vi "PhiCorrect_RAW.vi"(1 "PhiCorrect_RAW":i16=773, 2 "RAW cmds 2D in":i16[][](array[numeric])=[[-21913, -13120, -6560, 0, 4372, 4384, -21862, -1, -21913, -13120, -6560, 0, 4328, 4340, -21862, -1, -21913, -13120, -6560, 0, 4284, 4296, -21862, -1, -21913, -13120, -6560, 0, 4240, 4251, -21862, -1, -21913, -13120, -6560, 0, 4195, 4207, -21862, -1, -21913, -13120, -6560, 0, 4151, 4163, -21862, -1, -21913, -13120, -6560, 0, 4107, 4118, -21862, -1, -21913, -13120, -6560, 0, 4063, 4074, -21862, -1, -21913, -13120, -6560, 0, 4019, 4030, -21862, -1, -21913, -13120, -6560, 0, 3975, 3986, -21862, -1, -21913, -13120, -6560, 0, 3930, 3941, -21862, -1, -21913, -13120, -6560, 0, 3886, 3897, -21862, -1, -21913, -13120, -6560, 0, 3842, 3853, -21862, -1, -21913, -13120, -6560, 0, 3798, 3808, -21862, -1, -21913, -13120, -6560, 0, 3754, 3764, -21862, -1, -21913, -13120, -6560, 0, 3710, 3720, -21862, -1, -21913, -13120, -6560, 0, 3665, 3675, -21862, -1, -21913, -13120, -6560, 0, 3621, 3631, -21862, -1, -21913, -13120, -6560, 0, 3577, 3587, -21862, -1, -21913, -13120, -6560, 0, 3533, 3543, -21862, -1, -21913, -13120, -6560, 0, 3489, 3498, -21862, -1, -21913, -13120, -6560, 0, 3444, 3454, -21862, -1, -21913, -13120, -6560, 0, 3400, 3410, -21862, -1, -21913, -13120, -6560, 0, 3356, 3365, -21862, -1, -21913, -13120, -6560, 0, 3312, 3321, -21862, -1, -21913, -13120, -6560, 0, 3268, 3277, -21862, -1, -21913, -13120, -6560, 0, 3224, 3233, -21862, -1, -21913, -13120, -6560, 0, 3179, 3188, -21862, -1, -21913, -13120, -6560, 0, 3135, 3144, -21862, -1, -21913, -13120, -6560, 0, 3091, 3100, -21862, -1, -21913, -13120, -6560, 0, 3047, 3055, -21862, -1, -21913, -13120, -6560, 0, 3003, 3011, -21862, -1, -21913, -13120, -6560, 0, 2959, 2967, -21862, -1, -21913, -13120, -6560, 0, 2914, 2922, -21862, -1, -21913, -13120, -6560, 0, 2870, 2878, -21862, -1, -21913, -13120, -6560, 0, 2826, 2834, -21862, -1, -21913, -13120, -6560, 0, 2782, 2790, -21862, -1, -21913, -13120, -6560, 0, 2738, 2745, -21862, -1, -21913, -13120, -6560, 0, 2694, 2701, -21862, -1, -21913, -13120, -6560, 0, 2649, 2657, -21862, -1, -21913, -13120, -6560, 0, 2605, 2612, -21862, -1, -21913, -13120, -6560, 0, 2561, 2568, -21862, -1, -21913, -13120, -6560, 0, 2517, 2524, -21862, -1, -21913, -13120, -6560, 0, 2473, 2479, -21862, -1, -21913, -13120, -6560, 0, 2429, 2435, -21862, -1, -21913, -13120, -6560, 0, 2384, 2391, -21862, -1, -21913, -13120, -6560, 0, 2340, 2347, -21862, -1, -21913, -13120, -6560, 0, 2296, 2302, -21862, -1, -21913, -13120, -6560, 0, 2252, 2258, -21862, -1, -21913, -13120, -6560, 0, 2208, 2214, -21862, -1, -21913, -13120, -6560, 0, 2164, 2169, -21862, -1, -21913, -13120, -6560, 0, 2119, 2125, -21862, -1, -21913, -13120, -6560, 0, 2075, 2081, -21862, -1, -21913, -13120, -6560, 0, 2031, 2037, -21862, -1, -21913, -13120, -6560, 0, 1987, 1992, -21862, -1, -21913, -13120, -6560, 0, 1943, 1948, -21862, -1, -21913, -13120, -6560, 0, 1898, 1904, -21862, -1, -21913, -13120, -6560, 0, 1854, 1859, -21862, -1, -21913, -13120, -6560, 0, 1810, 1815, -21862, -1, -21913, -13120, -6560, 0, 1766, 1771, -21862, -1, -21913, -13120, -6560, 0, 1722, 1726, -21862, -1, -21913, -13120, -6560, 0, 1678, 1682, -21862, -1, -21913, -13120, -6560, 0, 1633, 1638, -21862, -1, -21913, -13120, -6560, 0, 1589, 1594, -21862, -1, -21913, -13120, -6560, 0, 1545, 1549, -21862, -1, -21913, -13120, -6560, 0, 1501, 1505, -21862, -1, -21913, -13120, -6560, 0, 1457, 1461, -21862, -1, -21913, -13120, -6560, 0, 1413, 1416, -21862, -1, -21913, -13120, -6560, 0, 1368, 1372, -21862, -1, -21913, -13120, -6560, 0, 1324, 1328, -21862, -1, -21913, -13120, -6560, 0, 1280, 1284, -21862, -1, -21913, -13120, -6560, 0, 1236, 1239, -21862, -1, -21913, -13120, -6560, 0, 1192, 1195, -21862, -1, -21913, -13120, -6560, 0, 1148, 1151, -21862, -1, -21913, -13120, -6560, 0, 1103, 1106, -21862, -1, -21913, -13120, -6560, 0, 1059, 1062, -21862, -1, -21913, -13120, -6560, 0, 1015, 1018, -21862, -1, -21913, -13120, -6560, 0, 971, 973, -21862, -1, -21913, -13120, -6560, 0, 927, 929, -21862, -1, -21913, -13120, -6560, 0, 883, 885, -21862, -1, -21913, -13120, -6560, 0, 838, 841, -21862, -1, -21913, -13120, -6560, 0, 794, 796, -21862, -1, -21913, -13120, -6560, 0, 750, 752, -21862, -1, -21913, -13120, -6560, 0, 706, 708, -21862, -1, -21913, -13120, -6560, 0, 662, 663, -21862, -1, -21913, -13120, -6560, 0, 618, 619, -21862, -1, -21913, -13120, -6560, 0, 573, 575, -21862, -1, -21913, -13120, -6560, 0, 529, 531, -21862, -1, -21913, -13120, -6560, 0, 485, 486, -21862, -1, -21913, -13120, -6560, 0, 441, 442, -21862, -1, -21913, -13120, -6560, 0, 397, 398, -21862, -1, -21913, -13120, -6560, 0, 352, 353, -21862, -1, -21913, -13120, -6560, 0, 308, 309, -21862, -1, -21913, -13120, -6560, 0, 264, 265, -21862, -1, -21913, -13120, -6560, 0, 220, 220, -21862, -1, -21913, -13120, -6560, 0, 176, 176, -21862, -1, -21913, -13120, -6560, 0, 132, 132, -21862, -1, -21913, -13120, -6560, 0, 87, 88, -21862, -1, -21913, -13120, -6560, 0, 43, 43, -21862, -1, -21913, -13120, -6560, 0, -1, -1, -21862, -1], [-1, -1, -7, -1, 0, 0, 0, 0, -1, -1, -7, -1, 0, 0, 0, 0, -1, -1, -7, -1, 0, 0, 0, 0, -1, -1, -7, -1, 0, 0, 0, 0, -1, -1, -7, -1, 0, 0, 0, 0, -1, -1, -7, -1, 0, 0, 0, 0, -1, -1, -7, -1, 0, 0, 0, 0, -1, -1, -7, -1, 0, 0, 0, 0, -1, -1, -7, -1, 0, 0, 0, 0, -1, -1, -7, -1, 0, 0, 0, 0, -1, -1, -7, -1, 0, 0, 0, 0, -1, -1, -7, -1, 0, 0, 0, 0, -1, -1, -7, -1, 0, 0, 0, 0, -1, -1, -7, -1, 0, 0, 0, 0, -1, -1, -7, -1, 0, 0, 0, 0, -1, -1, -7, -1, 0, 0, 0, 0, -1, -1, -7, -1, 0, 0, 0, 0, -1, -1, -7, -1, 0, 0, 0, 0, -1, -1, -7, -1, 0, 0, 0, 0, -1, -1, -7, -1, 0, 0, 0, 0, -1, -1, -7, -1, 0, 0, 0, 0, -1, -1, -7, -1, 0, 0, 0, 0, -1, -1, -7, -1, 0, 0, 0, 0, -1, -1, -7, -1, 0, 0, 0, 0, -1, -1, -7, -1, 0, 0, 0, 0, -1, -1, -7, -1, 0, 0, 0, 0, -1, -1, -7, -1, 0, 0, 0, 0, -1, -1, -7, -1, 0, 0, 0, 0, -1, -1, -7, -1, 0, 0, 0, 0, -1, -1, -7, -1, 0, 0, 0, 0, -1, -1, -7, -1, 0, 0, 0, 0, -1, -1, -7, -1, 0, 0, 0, 0, -1, -1, -7, -1, 0, 0, 0, 0, -1, -1, -7, -1, 0, 0, 0, 0, -1, -1, -7, -1, 0, 0, 0, 0, -1, -1, -7, -1, 0, 0, 0, 0, -1, -1, -7, -1, 0, 0, 0, 0, -1, -1, -7, -1, 0, 0, 0, 0, -1, -1, -7, -1, 0, 0, 0, 0, -1, -1, -7, -1, 0, 0, 0, 0, -1, -1, -7, -1, 0, 0, 0, 0, -1, -1, -7, -1, 0, 0, 0, 0, -1, -1, -7, -1, 0, 0, 0, 0, -1, -1, -7, -1, 0, 0, 0, 0, -1, -1, -7, -1, 0, 0, 0, 0, -1, -1, -7, -1, 0, 0, 0, 0, -1, -1, -7, -1, 0, 0, 0, 0, -1, -1, -7, -1, 0, 0, 0, 0, -1, -1, -7, -1, 0, 0, 0, 0, -1, -1, -7, -1, 0, 0, 0, 0, -1, -1, -7, -1, 0, 0, 0, 0, -1, -1, -7, -1, 0, 0, 0, 0, -1, -1, -7, -1, 0, 0, 0, 0, -1, -1, -7, -1, 0, 0, 0, 0, -1, -1, -7, -1, 0, 0, 0, 0, -1, -1, -7, -1, 0, 0, 0, 0, -1, -1, -7, -1, 0, 0, 0, 0, -1, -1, -7, -1, 0, 0, 0, 0, -1, -1, -7, -1, 0, 0, 0, 0, -1, -1, -7, -1, 0, 0, 0, 0, -1, -1, -7, -1, 0, 0, 0, 0, -1, -1, -7, -1, 0, 0, 0, 0, -1, -1, -7, -1, 0, 0, 0, 0, -1, -1, -7, -1, 0, 0, 0, 0, -1, -1, -7, -1, 0, 0, 0, 0, -1, -1, -7, -1, 0, 0, 0, 0, -1, -1, -7, -1, 0, 0, 0, 0, -1, -1, -7, -1, 0, 0, 0, 0, -1, -1, -7, -1, 0, 0, 0, 0, -1, -1, -7, -1, 0, 0, 0, 0, -1, -1, -7, -1, 0, 0, 0, 0, -1, -1, -7, -1, 0, 0, 0, 0, -1, -1, -7, -1, 0, 0, 0, 0, -1, -1, -7, -1, 0, 0, 0, 0, -1, -1, -7, -1, 0, 0, 0, 0, -1, -1, -7, -1, 0, 0, 0, 0, -1, -1, -7, -1, 0, 0, 0, 0, -1, -1, -7, -1, 0, 0, 0, 0, -1, -1, -7, -1, 0, 0, 0, 0, -1, -1, -7, -1, 0, 0, 0, 0, -1, -1, -7, -1, 0, 0, 0, 0, -1, -1, -7, -1, 0, 0, 0, 0, -1, -1, -7, -1, 0, 0, 0, 0, -1, -1, -7, -1, 0, 0, 0, 0, -1, -1, -7, -1, 0, 0, 0, 0, -1, -1, -7, -1, 0, 0, 0, 0, -1, -1, -7, -1, 0, 0, 0, 0, -1, -1, -7, -1, 0, 0, 0, 0, -1, -1, -7, -1, 0, 0, 0, 0, -1, -1, -7, -1, 0, 0, 0, 0, -1, -1, -7, -1, 0, 0, 0, 0, -1, -1, -7, -1, 0, 0, 0, 0, -1, -1, -7, -1, 0, 0, 0, 0, -1, -1, -7, -1, 0, 0, 0, 0, -1, -1, -7, -1, 0, 0, 0, 0, -1, -1, -7, -1, 0, 0, 0, 0, -1, -1, -7, -1, 0, 0, 0, 0, -1, -1, -7, -1, 0, 0, 0, 0, -1, -1, -7, -1, 0, 0, 0, 0, -1, -1, -7, -1, 0, 0, 0, 0]]) -> (0 "RAW cmds 2D out":i16[][](array[numeric])=[[-21913, -13120, -6560, 0, 4372, 4384, -21862, -1, -21913, -13120, -6560, 0, 4328, 4340, -21862, -1, -21913, -13120, -6560, 0, 4284, 4296, -21862, -1, -21913, -13120, -6560, 0, 4240, 4251, -21862, -1, -21913, -13120, -6560, 0, 4195, 4207, -21862, -1, -21913, -13120, -6560, 0, 4151, 4163, -21862, -1, -21913, -13120, -6560, 0, 4107, 4118, -21862, -1, -21913, -13120, -6560, 0, 4063, 4074, -21862, -1, -21913, -13120, -6560, 0, 4019, 4030, -21862, -1, -21913, -13120, -6560, 0, 3975, 3986, -21862, -1, -21913, -13120, -6560, 0, 3930, 3941, -21862, -1, -21913, -13120, -6560, 0, 3886, 3897, -21862, -1, -21913, -13120, -6560, 0, 3842, 3853, -21862, -1, -21913, -13120, -6560, 0, 3798, 3808, -21862, -1, -21913, -13120, -6560, 0, 3754, 3764, -21862, -1, -21913, -13120, -6560, 0, 3710, 3720, -21862, -1, -21913, -13120, -6560, 0, 3665, 3675, -21862, -1, -21913, -13120, -6560, 0, 3621, 3631, -21862, -1, -21913, -13120, -6560, 0, 3577, 3587, -21862, -1, -21913, -13120, -6560, 0, 3533, 3543, -21862, -1, -21913, -13120, -6560, 0, 3489, 3498, -21862, -1, -21913, -13120, -6560, 0, 3444, 3454, -21862, -1, -21913, -13120, -6560, 0, 3400, 3410, -21862, -1, -21913, -13120, -6560, 0, 3356, 3365, -21862, -1, -21913, -13120, -6560, 0, 3312, 3321, -21862, -1, -21913, -13120, -6560, 0, 3268, 3277, -21862, -1, -21913, -13120, -6560, 0, 3224, 3233, -21862, -1, -21913, -13120, -6560, 0, 3179, 3188, -21862, -1, -21913, -13120, -6560, 0, 3135, 3144, -21862, -1, -21913, -13120, -6560, 0, 3091, 3100, -21862, -1, -21913, -13120, -6560, 0, 3047, 3055, -21862, -1, -21913, -13120, -6560, 0, 3003, 3011, -21862, -1, -21913, -13120, -6560, 0, 2959, 2967, -21862, -1, -21913, -13120, -6560, 0, 2914, 2922, -21862, -1, -21913, -13120, -6560, 0, 2870, 2878, -21862, -1, -21913, -13120, -6560, 0, 2826, 2834, -21862, -1, -21913, -13120, -6560, 0, 2782, 2790, -21862, -1, -21913, -13120, -6560, 0, 2738, 2745, -21862, -1, -21913, -13120, -6560, 0, 2694, 2701, -21862, -1, -21913, -13120, -6560, 0, 2649, 2657, -21862, -1, -21913, -13120, -6560, 0, 2605, 2612, -21862, -1, -21913, -13120, -6560, 0, 2561, 2568, -21862, -1, -21913, -13120, -6560, 0, 2517, 2524, -21862, -1, -21913, -13120, -6560, 0, 2473, 2479, -21862, -1, -21913, -13120, -6560, 0, 2429, 2435, -21862, -1, -21913, -13120, -6560, 0, 2384, 2391, -21862, -1, -21913, -13120, -6560, 0, 2340, 2347, -21862, -1, -21913, -13120, -6560, 0, 2296, 2302, -21862, -1, -21913, -13120, -6560, 0, 2252, 2258, -21862, -1, -21913, -13120, -6560, 0, 2208, 2214, -21862, -1, -21913, -13120, -6560, 0, 2164, 2169, -21862, -1, -21913, -13120, -6560, 0, 2119, 2125, -21862, -1, -21913, -13120, -6560, 0, 2075, 2081, -21862, -1, -21913, -13120, -6560, 0, 2031, 2037, -21862, -1, -21913, -13120, -6560, 0, 1987, 1992, -21862, -1, -21913, -13120, -6560, 0, 1943, 1948, -21862, -1, -21913, -13120, -6560, 0, 1898, 1904, -21862, -1, -21913, -13120, -6560, 0, 1854, 1859, -21862, -1, -21913, -13120, -6560, 0, 1810, 1815, -21862, -1, -21913, -13120, -6560, 0, 1766, 1771, -21862, -1, -21913, -13120, -6560, 0, 1722, 1726, -21862, -1, -21913, -13120, -6560, 0, 1678, 1682, -21862, -1, -21913, -13120, -6560, 0, 1633, 1638, -21862, -1, -21913, -13120, -6560, 0, 1589, 1594, -21862, -1, -21913, -13120, -6560, 0, 1545, 1549, -21862, -1, -21913, -13120, -6560, 0, 1501, 1505, -21862, -1, -21913, -13120, -6560, 0, 1457, 1461, -21862, -1, -21913, -13120, -6560, 0, 1413, 1416, -21862, -1, -21913, -13120, -6560, 0, 1368, 1372, -21862, -1, -21913, -13120, -6560, 0, 1324, 1328, -21862, -1, -21913, -13120, -6560, 0, 1280, 1284, -21862, -1, -21913, -13120, -6560, 0, 1236, 1239, -21862, -1, -21913, -13120, -6560, 0, 1192, 1195, -21862, -1, -21913, -13120, -6560, 0, 1148, 1151, -21862, -1, -21913, -13120, -6560, 0, 1103, 1106, -21862, -1, -21913, -13120, -6560, 0, 1059, 1062, -21862, -1, -21913, -13120, -6560, 0, 1015, 1018, -21862, -1, -21913, -13120, -6560, 0, 971, 973, -21862, -1, -21913, -13120, -6560, 0, 927, 929, -21862, -1, -21913, -13120, -6560, 0, 883, 885, -21862, -1, -21913, -13120, -6560, 0, 838, 841, -21862, -1, -21913, -13120, -6560, 0, 794, 796, -21862, -1, -21913, -13120, -6560, 0, 750, 752, -21862, -1, -21913, -13120, -6560, 0, 706, 708, -21862, -1, -21913, -13120, -6560, 0, 662, 663, -21862, -1, -21913, -13120, -6560, 0, 618, 619, -21862, -1, -21913, -13120, -6560, 0, 573, 575, -21862, -1, -21913, -13120, -6560, 0, 529, 531, -21862, -1, -21913, -13120, -6560, 0, 485, 486, -21862, -1, -21913, -13120, -6560, 0, 441, 442, -21862, -1, -21913, -13120, -6560, 0, 397, 398, -21862, -1, -21913, -13120, -6560, 0, 352, 353, -21862, -1, -21913, -13120, -6560, 0, 308, 309, -21862, -1, -21913, -13120, -6560, 0, 264, 265, -21862, -1, -21913, -13120, -6560, 0, 220, 220, -21862, -1, -21913, -13120, -6560, 0, 176, 176, -21862, -1, -21913, -13120, -6560, 0, 132, 132, -21862, -1, -21913, -13120, -6560, 0, 87, 88, -21862, -1, -21913, -13120, -6560, 0, 43, 43, -21862, -1, -21913, -13120, -6560, 0, -1, -1, -21862, -1], [-1, -1, -7, -1, 0, 0, 0, 773, -1, -1, -7, -1, 0, 0, 0, 773, -1, -1, -7, -1, 0, 0, 0, 773, -1, -1, -7, -1, 0, 0, 0, 773, -1, -1, -7, -1, 0, 0, 0, 773, -1, -1, -7, -1, 0, 0, 0, 773, -1, -1, -7, -1, 0, 0, 0, 773, -1, -1, -7, -1, 0, 0, 0, 773, -1, -1, -7, -1, 0, 0, 0, 773, -1, -1, -7, -1, 0, 0, 0, 773, -1, -1, -7, -1, 0, 0, 0, 773, -1, -1, -7, -1, 0, 0, 0, 773, -1, -1, -7, -1, 0, 0, 0, 773, -1, -1, -7, -1, 0, 0, 0, 773, -1, -1, -7, -1, 0, 0, 0, 773, -1, -1, -7, -1, 0, 0, 0, 773, -1, -1, -7, -1, 0, 0, 0, 773, -1, -1, -7, -1, 0, 0, 0, 773, -1, -1, -7, -1, 0, 0, 0, 773, -1, -1, -7, -1, 0, 0, 0, 773, -1, -1, -7, -1, 0, 0, 0, 773, -1, -1, -7, -1, 0, 0, 0, 773, -1, -1, -7, -1, 0, 0, 0, 773, -1, -1, -7, -1, 0, 0, 0, 773, -1, -1, -7, -1, 0, 0, 0, 773, -1, -1, -7, -1, 0, 0, 0, 773, -1, -1, -7, -1, 0, 0, 0, 773, -1, -1, -7, -1, 0, 0, 0, 773, -1, -1, -7, -1, 0, 0, 0, 773, -1, -1, -7, -1, 0, 0, 0, 773, -1, -1, -7, -1, 0, 0, 0, 773, -1, -1, -7, -1, 0, 0, 0, 773, -1, -1, -7, -1, 0, 0, 0, 773, -1, -1, -7, -1, 0, 0, 0, 773, -1, -1, -7, -1, 0, 0, 0, 773, -1, -1, -7, -1, 0, 0, 0, 773, -1, -1, -7, -1, 0, 0, 0, 773, -1, -1, -7, -1, 0, 0, 0, 773, -1, -1, -7, -1, 0, 0, 0, 773, -1, -1, -7, -1, 0, 0, 0, 773, -1, -1, -7, -1, 0, 0, 0, 773, -1, -1, -7, -1, 0, 0, 0, 773, -1, -1, -7, -1, 0, 0, 0, 773, -1, -1, -7, -1, 0, 0, 0, 773, -1, -1, -7, -1, 0, 0, 0, 773, -1, -1, -7, -1, 0, 0, 0, 773, -1, -1, -7, -1, 0, 0, 0, 773, -1, -1, -7, -1, 0, 0, 0, 773, -1, -1, -7, -1, 0, 0, 0, 773, -1, -1, -7, -1, 0, 0, 0, 773, -1, -1, -7, -1, 0, 0, 0, 773, -1, -1, -7, -1, 0, 0, 0, 773, -1, -1, -7, -1, 0, 0, 0, 773, -1, -1, -7, -1, 0, 0, 0, 773, -1, -1, -7, -1, 0, 0, 0, 773, -1, -1, -7, -1, 0, 0, 0, 773, -1, -1, -7, -1, 0, 0, 0, 773, -1, -1, -7, -1, 0, 0, 0, 773, -1, -1, -7, -1, 0, 0, 0, 773, -1, -1, -7, -1, 0, 0, 0, 773, -1, -1, -7, -1, 0, 0, 0, 773, -1, -1, -7, -1, 0, 0, 0, 773, -1, -1, -7, -1, 0, 0, 0, 773, -1, -1, -7, -1, 0, 0, 0, 773, -1, -1, -7, -1, 0, 0, 0, 773, -1, -1, -7, -1, 0, 0, 0, 773, -1, -1, -7, -1, 0, 0, 0, 773, -1, -1, -7, -1, 0, 0, 0, 773, -1, -1, -7, -1, 0, 0, 0, 773, -1, -1, -7, -1, 0, 0, 0, 773, -1, -1, -7, -1, 0, 0, 0, 773, -1, -1, -7, -1, 0, 0, 0, 773, -1, -1, -7, -1, 0, 0, 0, 773, -1, -1, -7, -1, 0, 0, 0, 773, -1, -1, -7, -1, 0, 0, 0, 773, -1, -1, -7, -1, 0, 0, 0, 773, -1, -1, -7, -1, 0, 0, 0, 773, -1, -1, -7, -1, 0, 0, 0, 773, -1, -1, -7, -1, 0, 0, 0, 773, -1, -1, -7, -1, 0, 0, 0, 773, -1, -1, -7, -1, 0, 0, 0, 773, -1, -1, -7, -1, 0, 0, 0, 773, -1, -1, -7, -1, 0, 0, 0, 773, -1, -1, -7, -1, 0, 0, 0, 773, -1, -1, -7, -1, 0, 0, 0, 773, -1, -1, -7, -1, 0, 0, 0, 773, -1, -1, -7, -1, 0, 0, 0, 773, -1, -1, -7, -1, 0, 0, 0, 773, -1, -1, -7, -1, 0, 0, 0, 773, -1, -1, -7, -1, 0, 0, 0, 773, -1, -1, -7, -1, 0, 0, 0, 773, -1, -1, -7, -1, 0, 0, 0, 773, -1, -1, -7, -1, 0, 0, 0, 773, -1, -1, -7, -1, 0, 0, 0, 773, -1, -1, -7, -1, 0, 0, 0, 773, -1, -1, -7, -1, 0, 0, 0, 773, -1, -1, -7, -1, 0, 0, 0, 773, -1, -1, -7, -1, 0, 0, 0, 773, -1, -1, -7, -1, 0, 0, 0, 773, -1, -1, -7, -1, 0, 0, 0, 773]])   [LabVIEW 2018]
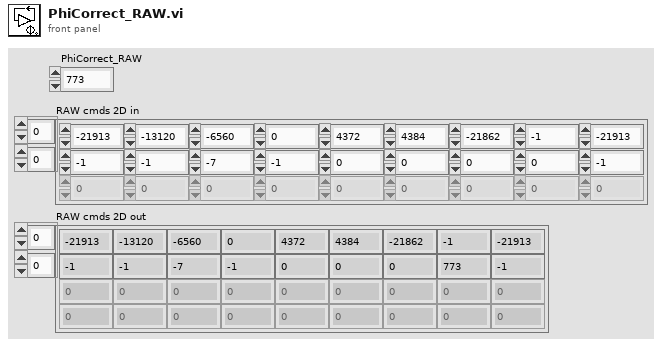
[diagram p1: front panel]
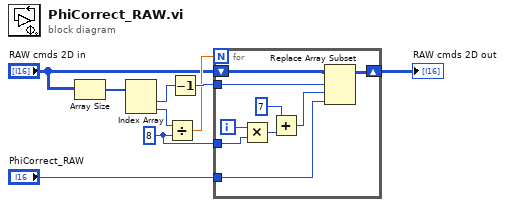
[diagram p0: block diagram]
diagram:
  w4 = 8 ("y")
  n1 = Array Size(array="RAW cmds 2D in") -> (size(s)=w7:i32[])
  n2 = Index Array(array=w7) -> (element #1=w9:i32, element #2=w6:i32)  [unwired: 2 in]
  n3 = Divide(x=w6, y=w4) -> (x/y=w5:dbl)
  n4 = Decrement(x=w9) -> (x-1=w8:i32)
  n5 = for {
    N: w5 -> [_]
    shift-right: [w14] -> w1
    shift-left: "RAW cmds 2D in" -> [w18]
    tunnel: w4 -> [w16]
    tunnel: "PhiCorrect_RAW" -> [w15]
    tunnel: w8 -> [w13]
    i -> [w17]
    n6 = Multiply(x=w17, y=w16) -> (x*y=w12:i32)
    n7 = Add(x=7, y=w12) -> (x+y=w10:i32)
    n8 = Replace Array Subset(array=w18, new element=w15, index (row)=w13, index (col)=w10) -> (w14:i16[][])
  }
  "RAW cmds 2D out" <- w1
